vi "final.vi"() -> ()   [LabVIEW 2016]
uses:
  <vilib>/robotics/Controls/Compass Indicator/Compass Indicator.xctl
  <vilib>/robotics/Controls/Attitude Indicator/Attitude Indicator.xctl
  <vilib>/Instr/_visa.llb/VISA Configure Serial Port (Instr).vi
panel:
  out "Numeric":dbl
  out "TEAM NAME":string
  out "LONGITUDE":dbl(knob) scale=0.0..10000.0 scale format="%.2f"
  out "PACKAGE NUMBER 2":dbl
  in  "stop":bool
  out "Intern String":string
  out "array":string[](array[string])
  out "ALTITUDE":dbl(graph)
  out "TIME":dbl
  out "SATELITE NUMBER":dbl
  out "PRESSURE":dbl(slide) scale=0.0..250.0
  out "LATITUDE":dbl(knob) scale=0.0..10000.0 scale format="%.2f"
  out "HEIGHT":dbl[](graph)
  out "ANGEL Z":dbl
  out "ACCELERATE Z":dbl
  out "ANGEL Y":dbl
  out "ACCELERATE Y":dbl
  out "ANGEL X":dbl
  out "ACCELERATE X":dbl
  out "HUMIDITY":dbl(slide) scale=0.0..100.0
  out "ACCELERATE  Y":dbl(knob) scale=0.0..5.0
  out "ACCELERATE  X":dbl(knob) scale=0.0..5.0
  out "ACCELERATE  Z":dbl(knob) scale=0.0..5.0
  out "ROLL & PITCH":cluster{"Roll":dbl, "Pitch":dbl}(xcontrol)
  out "AZIMUTH":dbl(xcontrol)
  out "ENVIROMENT TEMPRETURE":dbl(knob) scale=0.0..50.0
  out "LOWER FLOOR TEMPRETURE":dbl(slide) scale=0.0..50.0
  out "UPPER FLOOR TEMPRETURE":dbl(slide) scale=0.0..50.0
  out "SPEED":dbl(knob) scale=0.0..3.0
  out "LATITUDE DIRECTION":string
  in  "Stop Button":bool
  in  "milliseconds to wait":u32
  in  "OK Button":bool
  in  "VISA resource name":refnum<visa-resource-name>
  out "LONGITUDE DIRECTION":string
  # "PRIMARY CONFIGURATION"
  # "G"
  # "G"
  # "G"
  # "KM/H"
  # "DEGREE"
  # "DEGREE"
  # "DEGREE"
  # "DEGREE"
  # "KPA"
  # "%"
  # "G"
  # "in degree"
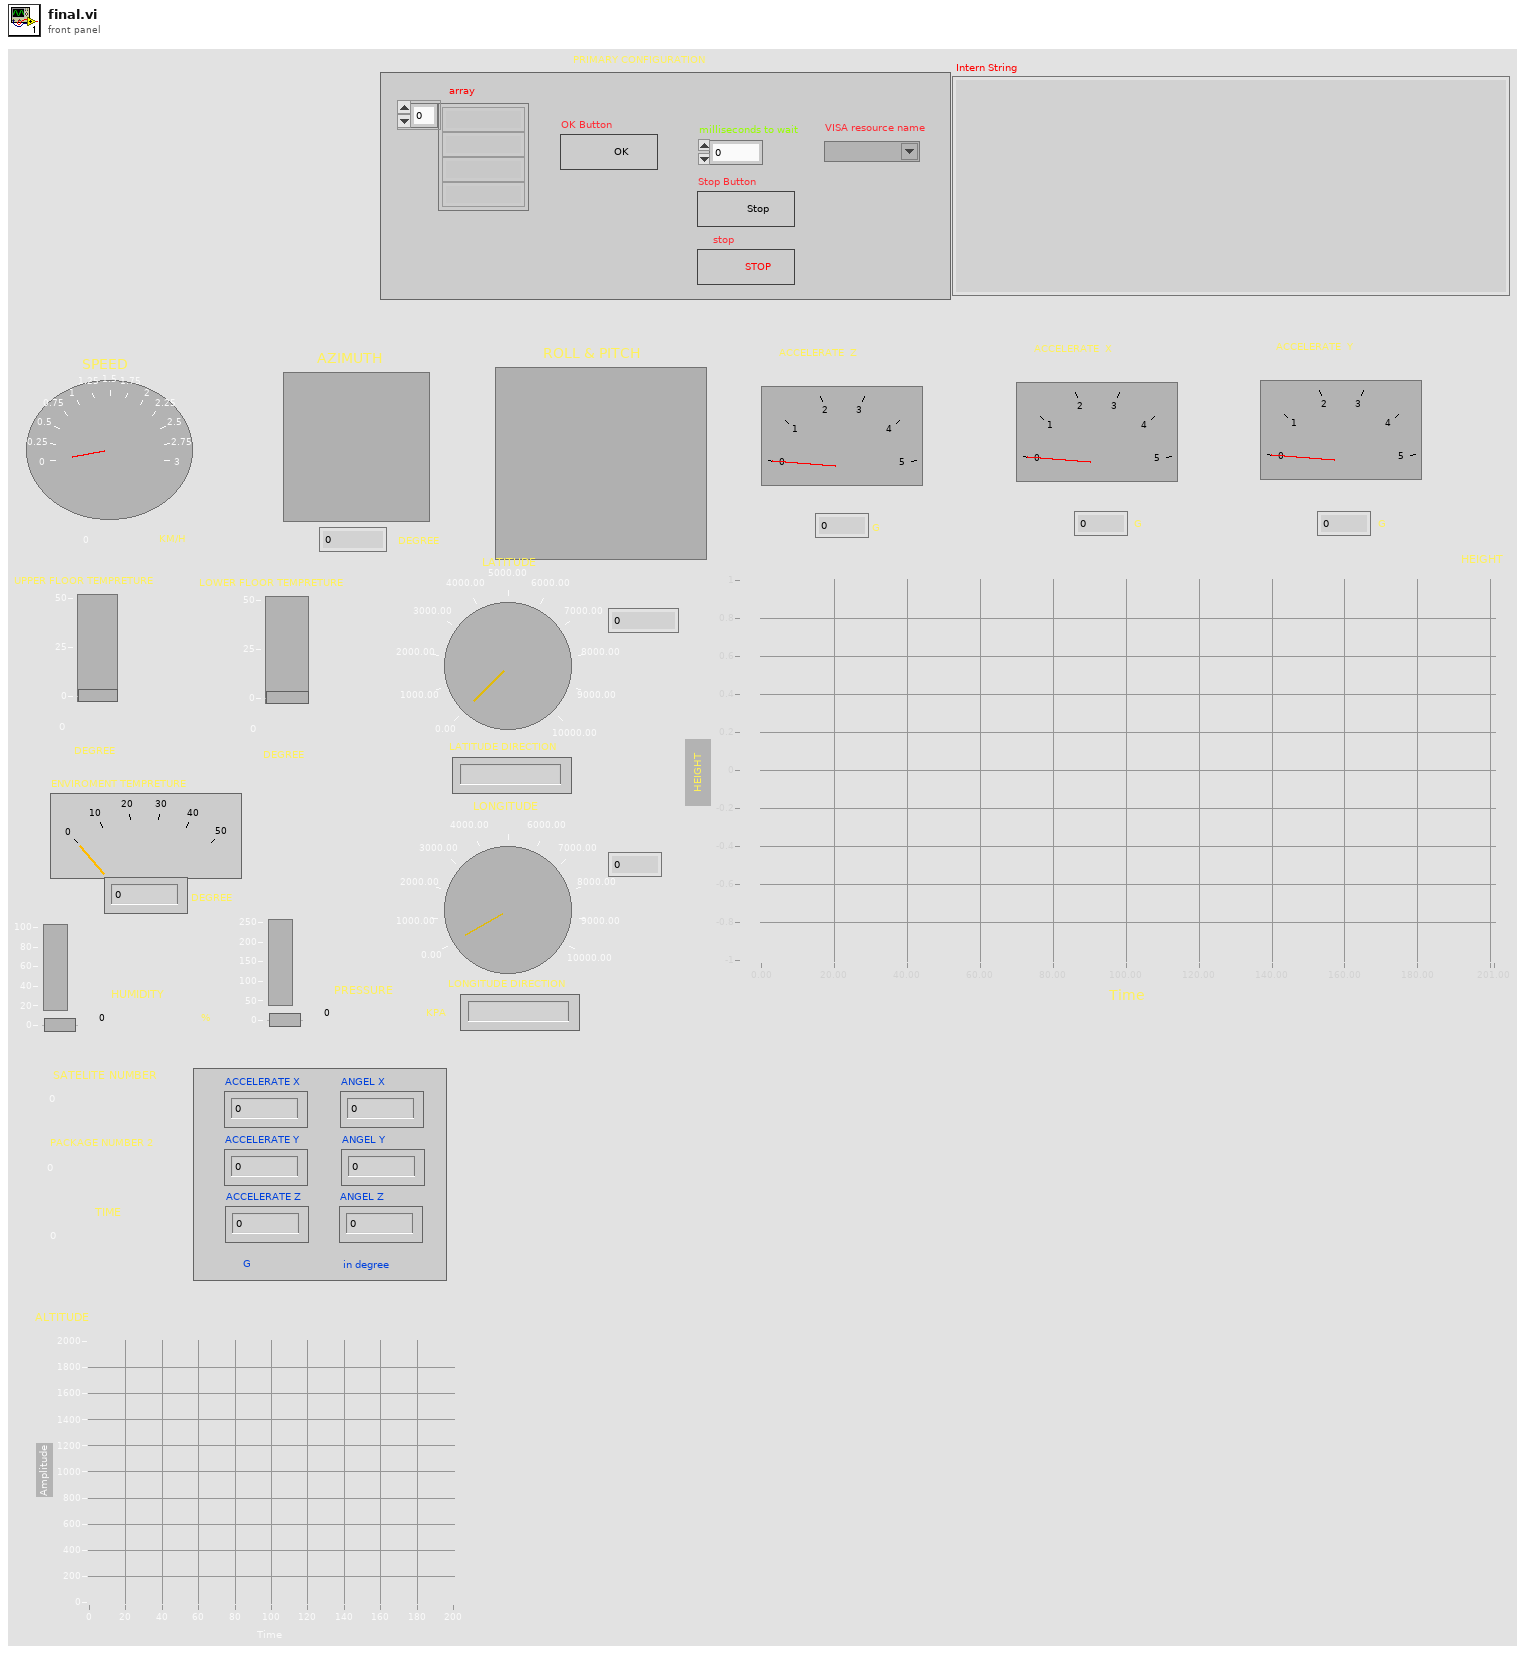
[diagram p1: front panel]
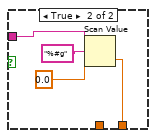
[diagram p3: hidden frame]
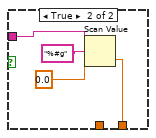
[diagram p4: hidden frame]
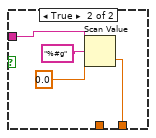
[diagram p5: hidden frame]
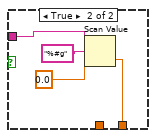
[diagram p7: hidden frame]
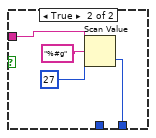
[diagram p8: hidden frame]
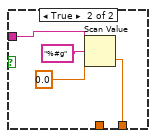
[diagram p9: hidden frame]
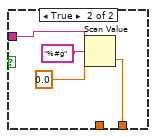
[diagram p10: hidden frame]
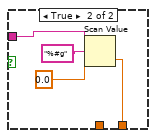
[diagram p11: hidden frame]
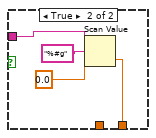
[diagram p12: hidden frame]
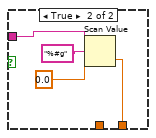
[diagram p13: hidden frame]
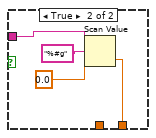
[diagram p14: hidden frame]
diagram:
  w3 = u16 0 items=["None", "XON/XOFF", "RTS/CTS", "XON/XOFF & RTS/CTS", "DTR/DSR", "XON/XOFF & DTR/DSR"] ("flow control (0:none)")
  w10 = u16 10 items=["1.0"=10, "1.5"=15, "2.0"=20] ("stop bits (10: 1 bit)")
  n1 = call-poly "VISA Configure Serial Port"("VISA resource name"="VISA resource name", "timeout (10sec)"=u32 10000, "termination char\n(0xA = '\\n' = LF)"=u8 10 ("termination char\n(0xA = '\\n' = LF)"), "Enable Termination\nChar (T)"=TRUE ("Enable Termination\nChar (T)"), "baud rate (9600)"=u32 14400, "data bits (8)"=u16 8, "parity (0:none)"=enum16{"None", "Odd", "Even", "Mark", "Space"}."None", "stop bits (10: 1 bit)"=w10, "flow control (0:none)"=w3) -> ("VISA resource name out"=w7:refnum<visa-resource-name>, "error out"=w6:errorcluster)  [unwired: 5 in]
  n2 = while {
    shift-right: [w21] -> w5
    shift-left: w7 -> [w23]
    tunnel: w6 -> [w22]
    tunnel: [w19] -> w4
    stop <- w20 stop-if-true
    n3 = Wait (ms)(milliseconds to wait="milliseconds to wait") -> ()  [unwired: 1 out]
    n4 = call "final (SubVI).vi"() -> ("SceneObject out"=w17:refnum<vi>)  [unwired: 11 in]
    n5 = case shown="True" "OK Button" {
      tunnel: w23 -> [_ w40]
      tunnel: w22 -> [_ w39]
      tunnel: [_ w35] -> w19
      tunnel: [_ w34] -> w21
      tunnel: w17 -> [_ w24]
      frame False {
      }
      frame True {
        n6 = property class="Instr"(reference=w40, error in=w39) -> (reference out=w38:refnum<visa-resource-name>, error out=w37:errorcluster, "Serial Settings:Number of Bytes at Serial Port"=w36:u32)
        n7 = VISA Read(VISA resource name=w38, byte count=w36, error in (no error)=w37) -> (VISA resource name out=w34:refnum<visa-resource-name>, read buffer=w30:string, error out=w35:errorcluster)  [unwired: 1 out]
        n8 = feedback #1("") -> (w32:string)
        n9 = Concatenate Strings(w32, w30) -> (w33:string)
        "Intern String" <- w33
        n10 = feedback-in #1(w33) -> ()
        n11 = Spreadsheet String To Array(delimiter (Tab)=",", format string="%s", spreadsheet string=w30, array type (2D Dbl)=string[] []) -> (array=w26:string[])
        "array" <- w26
        n12 = Array Size(array=w26) -> (size(s)=w25:i32)
        n13 = for {
          N: w25 -> [_]
          tunnel: w26 -> [w125]
          tunnel: w24 -> [w77]
          i -> [w124]
          # "speed"
          # "speed"
          # "speed"
          # "UPPER FLOOR TEMPRETURE"
          # "temprature ds18b20"
          # "satlite no"
          # "Azimuth"
          # "Altitude"
          # "accelerate Z"
          # "accelerate Y"
          # "accelerate X"
          # "angel Z"
          # "angel Y"
          # "angel x"
          # "humidity"
          # "pressure"
          # "ENVIROMENT TEMPRETURE"
          # "heigth"
          # "west"
          # "North"
          # "latitiude"
          # "package number"
          # "time"
          n14 = Index Array(array=w125, index=w124) -> (element=w123:string)
          n15 = Replace Substring(2:u8 1, 3:u8 0, 5:w123) -> (0:w54:string, 1:w44:string)  [unwired: 1 in]
          n16 = Equal?(x=w54, y="a") -> (x = y?=w132:bool)
          n17 = feedback #2() -> (w62:dbl)  [unwired: 1 in]
          "TIME" <- w62
          n18 = case shown="True" w132 {
            tunnel: w44 -> [_ w241]
            tunnel: [w239 w240] -> w129
            tunnel: w62 -> [w239 _]
            frame False {
            }
            frame True {
              n19 = Scan Value(string=w241, format string="%#g", default (0 dbl)=0.0) -> (value=w240:dbl)  [unwired: 1 out]
            }
          }
          n20 = feedback-in #2(w129) -> ()
          n21 = Equal?(x=w54, y="c") -> (x = y?=w128:bool)
          n22 = feedback #3() -> (w65:dbl)  [unwired: 1 in]
          "LATITUDE" <- w65
          n23 = case shown="True" w128 {
            tunnel: w44 -> [_ w236]
            tunnel: [w234 w235] -> w127
            tunnel: w65 -> [w234 _]
            frame False {
            }
            frame True {
              n24 = Scan Value(string=w236, format string="%#g", default (0 dbl)=0.0) -> (value=w235:dbl)  [unwired: 1 out]
            }
          }
          n25 = feedback-in #3(w127) -> ()
          n26 = Equal?(x=w54, y="d") -> (x = y?=w126:bool)
          n27 = case shown="True" w126 {
            tunnel: w44 -> [_ w231]
            frame False {
            }
            frame True {
              n28 = Scan Value(string=w231, format string="%#g", default (0 dbl)=0.0) -> (output string=→"LATITUDE DIRECTION":string)  [unwired: 1 out]
            }
          }
          n29 = Equal?(x=w54, y="f") -> (x = y?=w121:bool)
          n30 = case shown="True" w121 {
            tunnel: w44 -> [_ w227]
            frame False {
            }
            frame True {
              n31 = Scan Value(string=w227, format string="%#g", default (0 dbl)=0.0) -> (output string=→"LONGITUDE DIRECTION":string)  [unwired: 1 out]
            }
          }
          n32 = Equal?(x=w54, y="g") -> (x = y?=w119:bool)
          n33 = feedback #4() -> (w66:dbl)  [unwired: 1 in]
          n34 = case shown="True" w119 {
            tunnel: w44 -> [_ w223]
            tunnel: [w221 w222] -> w118
            tunnel: w66 -> [w221 _]
            frame False {
            }
            frame True {
              n35 = Scan Value(string=w223, format string="%#g", default (0 dbl)=0.0) -> (value=w222:dbl)  [unwired: 1 out]
            }
          }
          n36 = Build Array(w66) -> (→"HEIGHT":dbl[])
          n37 = feedback-in #4(w118) -> ()
          n38 = Equal?(x=w54, y="h") -> (x = y?=w116:bool)
          n39 = feedback #5() -> (w71:dbl)  [unwired: 1 in]
          "ENVIROMENT TEMPRETURE" <- w71
          n40 = case shown="True" w116 {
            tunnel: w44 -> [_ w218]
            tunnel: [w216 w217] -> w115
            tunnel: w71 -> [w216 _]
            frame False {
            }
            frame True {
              n41 = Scan Value(string=w218, format string="%#g", default (0 dbl)=0.0) -> (value=w217:dbl)  [unwired: 1 out]
            }
          }
          n42 = feedback-in #5(w115) -> ()
          n43 = Equal?(x=w54, y="i") -> (x = y?=w113:bool)
          n44 = feedback #6() -> (w64:dbl)  [unwired: 1 in]
          "PRESSURE" <- w64
          n45 = case shown="True" w113 {
            tunnel: w44 -> [_ w213]
            tunnel: [w211 w212] -> w112
            tunnel: w64 -> [w211 _]
            frame False {
            }
            frame True {
              n46 = Scan Value(string=w213, format string="%#g", default (0 dbl)=0.0) -> (value=w212:dbl)  [unwired: 1 out]
            }
          }
          n47 = feedback-in #6(w112) -> ()
          n48 = Equal?(x=w54, y="j") -> (x = y?=w110:bool)
          n49 = feedback #7() -> (w68:i32)  [unwired: 1 in]
          "HUMIDITY" <- w68
          n50 = case shown="True" w110 {
            tunnel: w44 -> [_ w208]
            tunnel: [w206 w207] -> w109
            tunnel: w68 -> [w206 _]
            frame False {
            }
            frame True {
              n51 = Scan Value(string=w208, format string="%#g", default (0 dbl)=35) -> (value=w207:i32)  [unwired: 1 out]
            }
          }
          n52 = feedback-in #7(w109) -> ()
          n53 = Equal?(x=w54, y="k") -> (x = y?=w107:bool)
          n54 = feedback #8() -> (w51:dbl)  [unwired: 1 in]
          "ANGEL X" <- w51
          n55 = case shown="True" w107 {
            tunnel: w44 -> [_ w203]
            tunnel: [w201 w202] -> w106
            tunnel: w51 -> [w201 _]
            frame False {
            }
            frame True {
              n56 = Scan Value(string=w203, format string="%#g", default (0 dbl)=0.0) -> (value=w202:dbl)  [unwired: 1 out]
            }
          }
          n57 = feedback-in #8(w106) -> ()
          n58 = Equal?(x=w54, y="l") -> (x = y?=w104:bool)
          n59 = feedback #9() -> (w50:dbl)  [unwired: 1 in]
          "ANGEL Y" <- w50
          n60 = Build Array(w51, w50) -> (w70:dbl[])
          n61 = Array To Cluster(array=w70) -> (cluster=→"ROLL & PITCH":cluster{"[0]":dbl, "[1]":dbl})
          n62 = call "final 2 (SubVI).vi"("Angel Y"=w50, "Angel x"=w51, "SceneObject in"=w77) -> ()  [unwired: 8 in, 1 out]
          n63 = case shown="True" w104 {
            tunnel: w44 -> [_ w198]
            tunnel: [w196 w197] -> w103
            tunnel: w50 -> [w196 _]
            frame False {
            }
            frame True {
              n64 = Scan Value(string=w198, format string="%#g", default (0 dbl)=0.0) -> (value=w197:dbl)  [unwired: 1 out]
            }
          }
          n65 = feedback-in #9(w103) -> ()
          n66 = Equal?(x=w54, y="m") -> (x = y?=w45:bool)
          n67 = feedback #10() -> (w43:dbl)  [unwired: 1 in]
          "ANGEL Z" <- w43
          n68 = case shown="False" w45 {
            tunnel: w44 -> [_ w138]
            tunnel: [w136 w137] -> w46
            tunnel: w43 -> [w136 _]
            frame False {
            }
            frame True {
              n69 = Scan Value(string=w138, format string="%#g", default (0 dbl)=0.0) -> (value=w137:dbl)  [unwired: 1 out]
            }
          }
          n70 = feedback-in #10(w46) -> ()
          n71 = Equal?(x=w54, y="n") -> (x = y?=w100:bool)
          n72 = feedback #11() -> (w49:dbl)  [unwired: 1 in]
          "ACCELERATE  X" <- w49
          "ACCELERATE X" <- w49
          n73 = case shown="False" w100 {
            tunnel: w44 -> [_ w193]
            tunnel: [w191 w192] -> w99
            tunnel: w49 -> [w191 _]
            frame False {
            }
            frame True {
              n74 = Scan Value(string=w193, format string="%#g", default (0 dbl)=0.0) -> (value=w192:dbl)  [unwired: 1 out]
            }
          }
          n75 = feedback-in #11(w99) -> ()
          n76 = Equal?(x=w54, y="o") -> (x = y?=w97:bool)
          n77 = feedback #12() -> (w48:dbl)  [unwired: 1 in]
          "ACCELERATE  Y" <- w48
          "ACCELERATE Y" <- w48
          n78 = case shown="False" w97 {
            tunnel: w44 -> [_ w188]
            tunnel: [w186 w187] -> w96
            tunnel: w48 -> [w186 _]
            frame False {
            }
            frame True {
              n79 = Scan Value(string=w188, format string="%#g", default (0 dbl)=0.0) -> (value=w187:dbl)  [unwired: 1 out]
            }
          }
          n80 = feedback-in #12(w96) -> ()
          n81 = Equal?(x=w54, y="p") -> (x = y?=w94:bool)
          n82 = feedback #13() -> (w47:dbl)  [unwired: 1 in]
          "ACCELERATE  Z" <- w47
          "ACCELERATE Z" <- w47
          n83 = case shown="False" w94 {
            tunnel: w44 -> [_ w183]
            tunnel: [w181 w182] -> w93
            tunnel: w47 -> [w181 _]
            frame False {
            }
            frame True {
              n84 = Scan Value(string=w183, format string="%#g", default (0 dbl)=0.0) -> (value=w182:dbl)  [unwired: 1 out]
            }
          }
          n85 = feedback-in #13(w93) -> ()
          n86 = Equal?(x=w54, y="q") -> (x = y?=w91:bool)
          n87 = feedback #14() -> (w61:dbl)  [unwired: 1 in]
          "ALTITUDE" <- w61
          n88 = case shown="False" w91 {
            tunnel: w44 -> [_ w178]
            tunnel: [w176 w177] -> w90
            tunnel: w61 -> [w176 _]
            frame False {
            }
            frame True {
              n89 = Scan Value(string=w178, format string="%#g", default (0 dbl)=0.0) -> (value=w177:dbl)  [unwired: 1 out]
            }
          }
          n90 = feedback-in #14(w90) -> ()
          n91 = Equal?(x=w54, y="r") -> (x = y?=w88:bool)
          n92 = feedback #15() -> (w41:dbl)  [unwired: 1 in]
          "AZIMUTH" <- w41
          "Numeric" <- w41
          n93 = case shown="False" w88 {
            tunnel: w44 -> [_ w173]
            tunnel: [w171 w172] -> w87
            tunnel: w41 -> [w171 _]
            frame False {
            }
            frame True {
              n94 = Scan Value(string=w173, format string="%#g", default (0 dbl)=0.0) -> (value=w172:dbl)  [unwired: 1 out]
            }
          }
          n95 = feedback-in #15(w87) -> ()
          n96 = Equal?(x=w54, y="s") -> (x = y?=w85:bool)
          n97 = feedback #16() -> (w63:dbl)  [unwired: 1 in]
          "SATELITE NUMBER" <- w63
          n98 = case shown="False" w85 {
            tunnel: w44 -> [_ w168]
            tunnel: [w166 w167] -> w84
            tunnel: w63 -> [w166 _]
            frame False {
            }
            frame True {
              n99 = Scan Value(string=w168, format string="%#g", default (0 dbl)=0.0) -> (value=w167:dbl)  [unwired: 1 out]
            }
          }
          n100 = feedback-in #16(w84) -> ()
          n101 = Equal?(x=w54, y="t") -> (x = y?=w82:bool)
          n102 = feedback #17() -> (w72:i32)  [unwired: 1 in]
          "LOWER FLOOR TEMPRETURE" <- w72
          n103 = case shown="False" w82 {
            tunnel: w44 -> [_ w163]
            tunnel: [w161 w162] -> w81
            tunnel: w72 -> [w161 _]
            frame False {
            }
            frame True {
              n104 = Scan Value(string=w163, format string="%#g", default (0 dbl)=27) -> (value=w162:i32)  [unwired: 1 out]
            }
          }
          n105 = feedback-in #17(w81) -> ()
          n106 = Equal?(x=w54, y="u") -> (x = y?=w79:bool)
          n107 = feedback #18() -> (w73:dbl)  [unwired: 1 in]
          "UPPER FLOOR TEMPRETURE" <- w73
          n108 = case shown="False" w79 {
            tunnel: w44 -> [_ w158]
            tunnel: [w156 w157] -> w78
            tunnel: w73 -> [w156 _]
            frame False {
            }
            frame True {
              n109 = Scan Value(string=w158, format string="%#g", default (0 dbl)=0.0) -> (value=w157:dbl)  [unwired: 1 out]
            }
          }
          n110 = feedback-in #18(w78) -> ()
          n111 = Equal?(x=w54, y="v") -> (x = y?=w75:bool)
          n112 = feedback #19() -> (w42:dbl)  [unwired: 1 in]
          "SPEED" <- w42
          n113 = case shown="True" w75 {
            tunnel: w44 -> [_ w153]
            tunnel: [w151 w152] -> w74
            tunnel: w42 -> [w151 _]
            frame False {
            }
            frame True {
              n114 = Scan Value(string=w153, format string="%#g", default (0 dbl)=0.0) -> (value=w152:dbl)  [unwired: 1 out]
            }
          }
          n115 = feedback-in #19(w74) -> ()
          n116 = Equal?(x=w54, y="b") -> (x = y?=w59:bool)
          n117 = feedback #20() -> (w53:dbl)  [unwired: 1 in]
          "PACKAGE NUMBER 2" <- w53
          n118 = case shown="False" w59 {
            tunnel: w44 -> [_ w148]
            tunnel: [w146 w147] -> w58
            tunnel: w53 -> [w146 _]
            frame False {
            }
            frame True {
              n119 = Scan Value(string=w148, format string="%#g", default (0 dbl)=0.0) -> (value=w147:dbl)  [unwired: 1 out]
            }
          }
          n120 = feedback-in #20(w58) -> ()
          n121 = Equal?(x=w54, y="e") -> (x = y?=w56:bool)
          n122 = feedback #21() -> (w52:dbl)  [unwired: 1 in]
          "LONGITUDE" <- w52
          n123 = case shown="False" w56 {
            tunnel: w44 -> [_ w143]
            tunnel: [w141 w142] -> w55
            tunnel: w52 -> [w141 _]
            frame False {
            }
            frame True {
              n124 = Scan Value(string=w143, format string="%#g", default (0 dbl)=0.0) -> (value=w142:dbl)  [unwired: 1 out]
            }
          }
          n125 = feedback-in #21(w55) -> ()
        }
      }
    }
    n126 = Or(x=w19, y="stop") -> (x .or. y?=w20:bool)
  }
  n127 = VISA Close(VISA resource name=w5, error in (no error)=w4) -> ()  [unwired: 1 out]
  "TEAM NAME" <- "  SUTECH SAT" ("TEAM NAME")
